vi "Follow.vi"() -> ()   [LabVIEW 2017]
uses:
  Robot Global Data.vi
panel:
  in  "Path Name":string
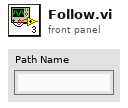
[diagram p1: front panel]
types:
  T1 = cluster{"WP#":i32, "Mode":string, "Power":dbl, "Heading":dbl, "Ramp_L":dbl, "Ramp_R":dbl, "End":dbl}[]
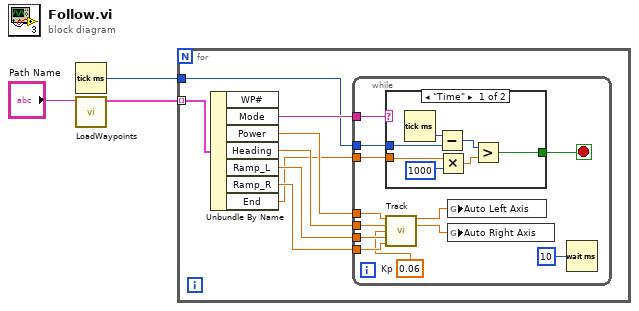
[diagram p0: block diagram]
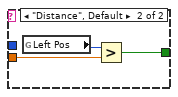
[diagram p2: hidden frame]
diagram:
  n1 = Tick Count (ms)() -> (millisecond timer value=w2:u32)
  n2 = call "LoadWaypoints.vi"("Path Name"="Path Name") -> ("Waypoints"=w3:T1)  [unwired: 10 in]
  n3 = for {
    tunnel: w3 -> [w11] mode=indexing
    tunnel: w2 -> [w9]
    n4 = Unbundle By Name(w11) -> ("Mode"=w10:string, "Power"=w8:dbl, "Heading"=w7:dbl, "Ramp_L"=w6:dbl, "Ramp_R"=w5:dbl, "End"=w4:dbl)  [unwired: 1 out]
    n5 = while {
      tunnel: w10 -> [w23]
      tunnel: w4 -> [w22]
      tunnel: w9 -> [w20]
      tunnel: w8 -> [w19]
      tunnel: w7 -> [w18]
      tunnel: w6 -> [w17]
      tunnel: w5 -> [w16]
      stop <- w21 stop-if-true
      w14 = 0.06  # Kp
      n6 = case shown="\"Time\"" w23 {
        tunnel: w22 -> [w24 w32]
        tunnel: [w27 w31] -> w21
        tunnel: w20 -> [w29 _]
        frame "Time" {
          n7 = Tick Count (ms)() -> (millisecond timer value=w30:u32)
          n8 = Subtract(x=w30, y=w29) -> (x-y=w28:u32)
          n9 = Multiply(x=w24, y=1000) -> (x*y=w26:dbl)
          n10 = Greater?(x=w28, y=w26) -> (0:w27:bool)
        }
        frame "Distance", Default {
          n11 = global read "Robot Global Data.vi" "Left Pos"() -> (w33:i32)
          n12 = Greater?(x=w33, y=w32) -> (0:w31:bool)
        }
      }
      n13 = call "Track.vi"("Power"=w19, "Heading"=w18, "Kp"=w14, "Ramp_L"=w17, "Ramp_R"=w16) -> ("Magnitude Left"=w13:dbl, "Magnitude Right"=w12:dbl)  [unwired: 7 in, 2 out]
      n14 = global write "Robot Global Data.vi" "Auto Left Axis"(w13) -> ()
      n15 = global write "Robot Global Data.vi" "Auto Right Axis"(w12) -> ()
      n16 = Wait (ms)(milliseconds to wait=10) -> ()  [unwired: 1 out]
    }
  }
